vi "Tabbed Subpanels.vi"() -> ()   [LabVIEW 2020, in "SubPanels.lvlib"]
uses:
  SubPanels.lvlib
  OOPanel/Manager/Manager.lvclass
  SubClone/SubClone.lvclass
panel:
  in  "Tab":enum32{"Page 1", "Page 2"}(tab)
  in  "G - A":bool
  in  "Y - A":bool
  in  "Out A":bool
  in  "X A":bool
  in  "G - B":bool
  in  "Y - B":bool
  in  "Out B":bool
  in  "X B":bool
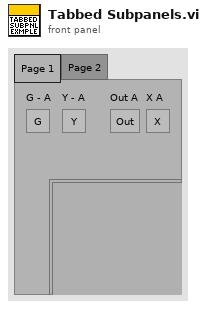
[diagram p1: front panel]
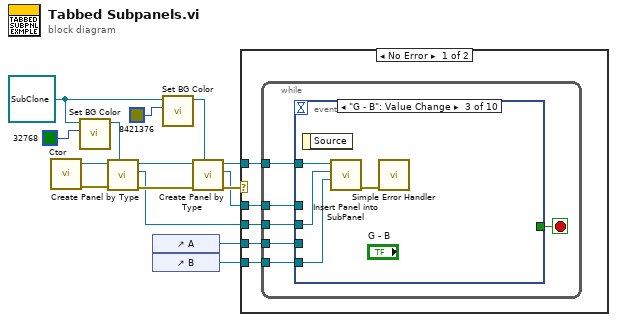
[diagram p0: block diagram]
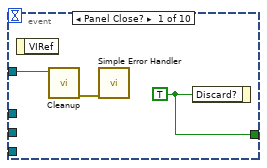
[diagram p2: hidden frame]
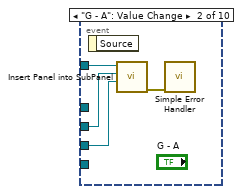
[diagram p3: hidden frame]
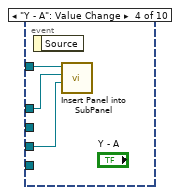
[diagram p4: hidden frame]
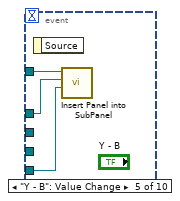
[diagram p5: hidden frame]
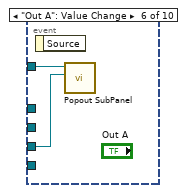
[diagram p6: hidden frame]
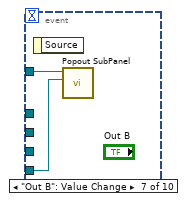
[diagram p7: hidden frame]
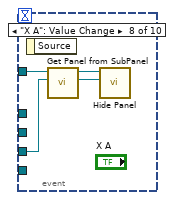
[diagram p8: hidden frame]
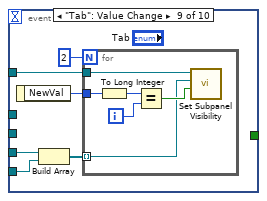
[diagram p9: hidden frame]
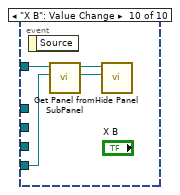
[diagram p10: hidden frame]
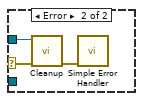
[diagram p11: hidden frame]
diagram:
  w2 = refnum<class "SubClone.lvclass"> refnum ("SubPanels.lvlib:SubClone.lvclass")
  n1 = call "Ctor.vi"() -> ("error out"=w1:errorcluster, "Manager out"=w10:refnum<class "Manager.lvclass">)  [unwired: 10 in]
  n2 = call "Set BG Color.vi"("BG"=u32 32768, "SubClone in"=w2) -> ("SubClone out"=w11:refnum<class "SubClone.lvclass">)  [unwired: 8 in, 1 out]
  n3 = call "Create Panel by Type.vi"("Panel Type"=w11, "error in (no error)"=w1, "Manager in"=w10) -> ("error out"=w14:errorcluster, "Panel"=w4:refnum<class "SubClone.lvclass">, "Manager out"=w9:refnum<class "Manager.lvclass">)  [unwired: 6 in]
  n4 = control-ref of="A"() -> (w6:refnum<vi>)
  n5 = control-ref of="B"() -> (w5:refnum<vi>)
  n6 = call "Set BG Color.vi"("BG"=u32 8421376, "SubClone in"=w2) -> ("SubClone out"=w8:refnum<class "SubClone.lvclass">)  [unwired: 8 in, 1 out]
  n7 = call "Create Panel by Type.vi"("Panel Type"=w8, "error in (no error)"=w14, "Manager in"=w9) -> ("error out"=w15:errorcluster, "Panel"=w3:refnum<class "SubClone.lvclass">, "Manager out"=w7:refnum<class "Manager.lvclass">)  [unwired: 6 in]
  n8 = case shown="No Error" w15 {
    selector: w15 -> [_ w69]
    tunnel: w7 -> [w20 w70]
    tunnel: w6 -> [w19 _]
    tunnel: w5 -> [w18 _]
    tunnel: w4 -> [w17 _]
    tunnel: w3 -> [w16 _]
    frame No Error {
      n9 = while {
        tunnel: w20 -> [w26]
        tunnel: w19 -> [w25]
        tunnel: w18 -> [w24]
        tunnel: w17 -> [w22]
        tunnel: w16 -> [w21]
        stop <- w23 stop-if-true
        n10 = event shown="[2] \"G - B\": Value Change" {
          selector: _ -> [_ _ _ _ _ _ _ _ _ _]
          dyn-events: _ -> [_ _ _ _ _ _ _ _ _ _]
          timeout: _ -> [_ _ _ _ _ _ _ _ _ _]
          tunnel: w26 -> [w28 w33 w37 w40 w43 w45 w47 w51 w52 w67]
          tunnel: w25 -> [_ w31 _ w38 _ w44 _ w50 w57 _]
          tunnel: w24 -> [_ _ w35 _ w42 _ w46 _ w56 w64]
          tunnel: [w29 _ _ _ _ _ _ _ _ _] -> w23
          tunnel: w22 -> [_ w32 w36 _ _ _ _ _ _ _]
          tunnel: w21 -> [_ _ _ w39 w41 _ _ _ _ _]
          event Panel Close? {
            w29 = TRUE ("Discard?")
            n11 = event-data() -> ()  [unwired: 1 in, 1 out]
            n12 = call "Cleanup.vi"("Manager in"=w28) -> ("error out"=w27:errorcluster)  [unwired: 8 in, 2 out]
            n13 = call <vilib>:"Simple Error Handler.vi"("error in (no error)"=w27) -> ()  [unwired: 4 in, 5 out]
            n14 = event-data("Discard?"=w29) -> ()  [unwired: 1 in, 1 out]
          }
          event "G - A": Value Change {
            n15 = event-data() -> ()  [unwired: 1 in, 1 out]
            n16 = call "Insert Panel into SubPanel.vi"("SubPanel"=w31, "Panel In"=w32, "Manager in"=w33) -> ("error out"=w30:errorcluster)  [unwired: 6 in, 2 out]
            n17 = call <vilib>:"Simple Error Handler.vi"("error in (no error)"=w30) -> ()  [unwired: 4 in, 5 out]
          }
          event "G - B": Value Change {
            n18 = event-data() -> ()  [unwired: 1 in, 1 out]
            n19 = call "Insert Panel into SubPanel.vi"("SubPanel"=w35, "Panel In"=w36, "Manager in"=w37) -> ("error out"=w34:errorcluster)  [unwired: 6 in, 2 out]
            n20 = call <vilib>:"Simple Error Handler.vi"("error in (no error)"=w34) -> ()  [unwired: 4 in, 5 out]
          }
          event "Y - A": Value Change {
            n21 = event-data() -> ()  [unwired: 1 in, 1 out]
            n22 = call "Insert Panel into SubPanel.vi"("SubPanel"=w38, "Panel In"=w39, "Manager in"=w40) -> ()  [unwired: 6 in, 3 out]
          }
          event "Y - B": Value Change {
            n23 = event-data() -> ()  [unwired: 1 in, 1 out]
            n24 = call "Insert Panel into SubPanel.vi"("SubPanel"=w42, "Panel In"=w41, "Manager in"=w43) -> ()  [unwired: 6 in, 3 out]
          }
          event "Out A": Value Change {
            n25 = event-data() -> ()  [unwired: 1 in, 1 out]
            n26 = call "Popout SubPanel.vi"("SubPanel"=w44, "Manager in"=w45) -> ()  [unwired: 8 in, 2 out]
          }
          event "Out B": Value Change {
            n27 = event-data() -> ()  [unwired: 1 in, 1 out]
            n28 = call "Popout SubPanel.vi"("SubPanel"=w46, "Manager in"=w47) -> ()  [unwired: 8 in, 2 out]
          }
          event "X A": Value Change {
            n29 = event-data() -> ()  [unwired: 1 in, 1 out]
            n30 = call "Get Panel from SubPanel.vi"("SubPanel"=w50, "Manager in"=w51) -> ("Panel"=w48:refnum<class "Panel.lvclass">, "Manager out"=w49:refnum<class "Manager.lvclass">)  [unwired: 6 in, 2 out]
            n31 = call "Hide Panel.vi"("Panel In"=w48, "Manager in"=w49) -> ()  [unwired: 7 in, 3 out]
          }
          event "Tab": Value Change {
            n32 = event-data() -> ("NewVal"=w53:enum32{"Page 1", "Page 2"})  [unwired: 1 in]
            n33 = Build Array(w57, w56) -> (w55:refnum<vi>[])
            n34 = for {
              N: 2 -> [_]
              tunnel: w55 -> [w58] mode=indexing
              tunnel: w53 -> [w63]
              tunnel: w52 -> [w60]
              i -> [w62]
              n35 = To Long Integer(number=w63) -> (32bit integer=w61:i32)
              n36 = Equal?(x=w61, y=w62) -> (x = y?=w59:bool)
              n37 = call "Set Subpanel Visibility.vi"("Visible"=w59, "SubPanel"=w58, "Manager in"=w60) -> ()  [unwired: 7 in, 2 out]
            }
          }
          event "X B": Value Change {
            n38 = event-data() -> ()  [unwired: 1 in, 1 out]
            n39 = call "Get Panel from SubPanel.vi"("SubPanel"=w64, "Manager in"=w67) -> ("Panel"=w65:refnum<class "Panel.lvclass">, "Manager out"=w66:refnum<class "Manager.lvclass">)  [unwired: 6 in, 2 out]
            n40 = call "Hide Panel.vi"("Panel In"=w65, "Manager in"=w66) -> ()  [unwired: 7 in, 3 out]
          }
        }
      }
    }
    frame Error {
      n41 = call "Cleanup.vi"("error in (no error)"=w69, "Manager in"=w70) -> ("error out"=w68:errorcluster)  [unwired: 7 in, 2 out]
      n42 = call <vilib>:"Simple Error Handler.vi"("error in (no error)"=w68) -> ()  [unwired: 4 in, 5 out]
    }
  }
